vi "temperatur_term_plot.vi"(10 "Enum":T1(ring)=enum."Celsius [C]", 11 "Numeric in":dbl) -> (2 "Waveform Chart 2":dbl(graph), 3 "Thermometer":dbl(slide) scale=-500.0..500.0)   [LabVIEW 2024]
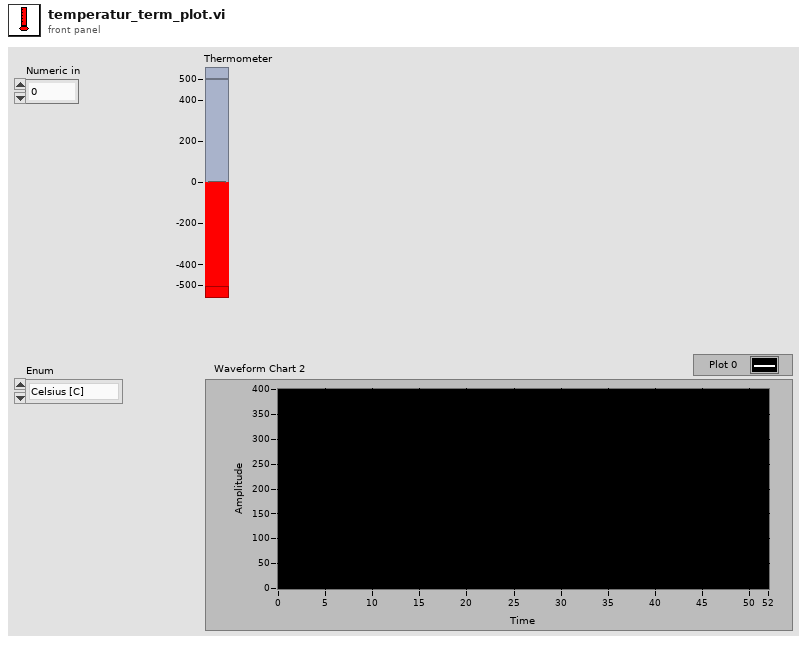
[diagram p1: front panel]
types:
  T1 = enum16{"Kelvin [K]", "Celsius [C]", "Fahrenheit [F]"}
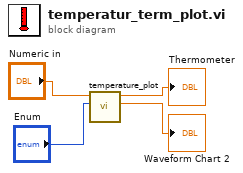
[diagram p0: block diagram]
diagram:
  n1 = call "temperature_plot.vi"("Enum"="Enum", "Numeric in"="Numeric in") -> ("Numeric 4"=→"Waveform Chart 2":dbl, "Numeric 3"=→"Thermometer":dbl)  [unwired: 8 in]
